vi "FunctionSelector.vi"(4 "System Control In":T2={"Start"=FALSE, "Stop"=FALSE, "Power System Enable"=FALSE, "SSG Control"=FALSE, "Virtual Inertia"=FALSE, "Manual Current"=FALSE, "Discharge"=FALSE, "Spot Generation"=FALSE, "Charge Control"=FALSE, "Watchdog"=FALSE, "ComAp Fault"=FALSE, "Clear Gen Faults"=FALSE, "Clear PV Faults"=FALSE, "Clear System Faults"=FALSE, "Clear PC Faults"=FALSE, "Clear ES Faults"=FALSE, "Clear Watchdog Faults"=FALSE, "PS V Setpoint"=0.0, "Manual Current"=0.0, "CC V Setpoint"=0.0, "Gen Capacity"=0.0, "Gen Reserve"=0.0, "VI gain P"=0.0, "CC gain P"=0.0, "Nom Hz"=0.0, "Spot Gen Op Value"=50.0, "CC gain I"=0.0, "CC Charge"=100.0, "CC Discharge"=-100.0, "Discharge Current"=-25.0, "Sign Of Life"=FALSE, "Reverse Rotation"=FALSE, "String Selector"=enum."3 Strings"}, 5 "Current Limit Parameters In":T4, 6 "Error In":errorcluster, 7 "FPGA Data":T1, 8 "VI Current In":dbl, 9 "CC Current In":dbl) -> (0 "Error Out":errorcluster, 2 "Current Out":dbl)   [LabVIEW 2013]
uses:
  eng/trunk/ni/cRIO Master Files/Controls/CurrentLimitParameters.ctl
  eng/trunk/ni/cRIO Master Files/Controls/SystemControl.ctl
  eng/trunk/ni/cRIO Master Files/Controls/StringSelector.ctl
  Controls/FPGAData.ctl
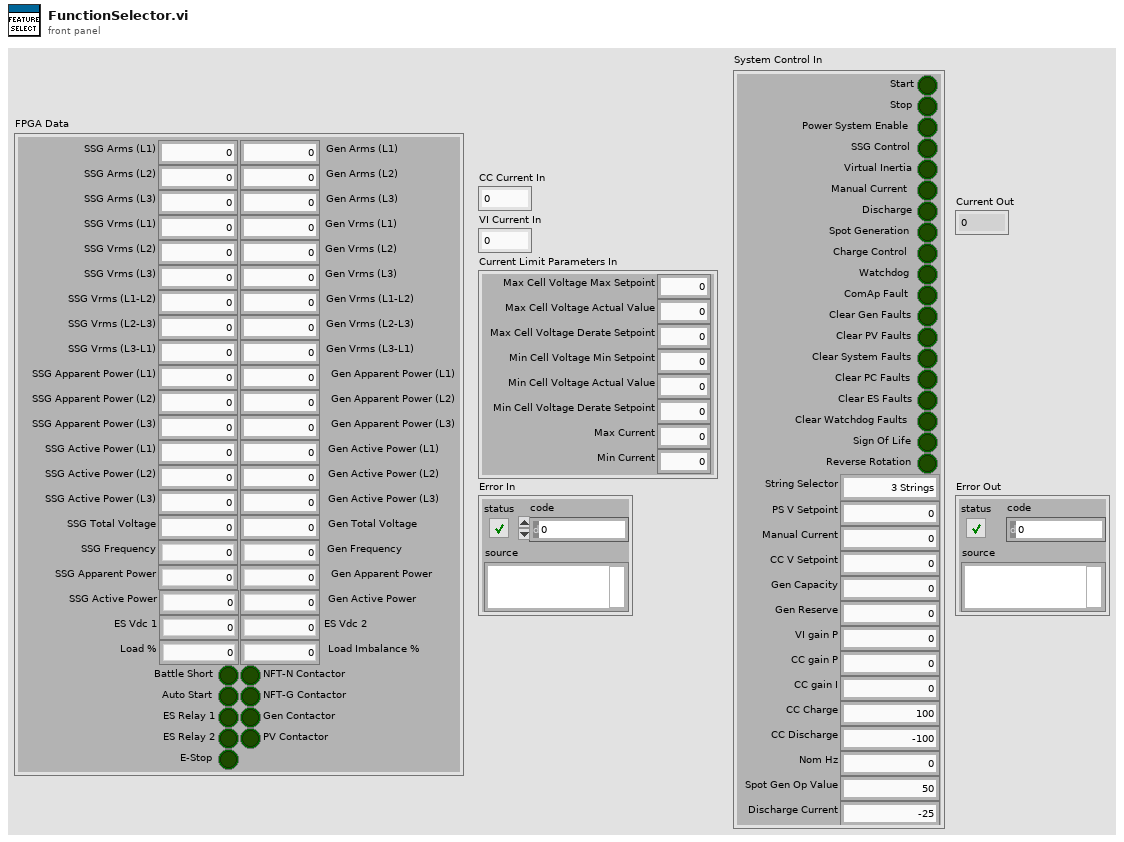
[diagram p1: front panel]
types:
  T1 = typedef "FPGAData.ctl" = cluster{"SSG Frequency":sgl, "SSG Total Voltage":dbl, "SSG Active Power":sgl, "SSG Apparent Power":sgl, "SSG Active Power (L1)":dbl, "SSG Active Power (L2)":dbl, "SSG Active Power (L3)":dbl, "SSG Apparent Power (L1)":dbl, "SSG Apparent Power (L2)":dbl, "SSG Apparent Power (L3)":dbl, "SSG Vrms (L1-L2)":dbl, "SSG Vrms (L2-L3)":dbl, "SSG Vrms (L3-L1)":dbl, "SSG Vrms (L1)":dbl, "SSG Vrms (L2)":dbl, "SSG Vrms (L3)":dbl, "SSG Arms (L1)":dbl, "SSG Arms (L2)":dbl, "SSG Arms (L3)":dbl, "Gen Frequency":sgl, "Gen Total Voltage":dbl, "Gen Active Power":sgl, "Gen Apparent Power":sgl, "Gen Active Power (L1)":dbl, "Gen Active Power (L2)":dbl, "Gen Active Power (L3)":dbl, "Gen Apparent Power (L1)":dbl, "Gen Apparent Power (L2)":dbl, "Gen Apparent Power (L3)":dbl, "Gen Vrms (L1-L2)":dbl, "Gen Vrms (L2-L3)":dbl, "Gen Vrms (L3-L1)":dbl, "Gen Vrms (L1)":dbl, "Gen Vrms (L2)":dbl, "Gen Vrms (L3)":dbl, "Gen Arms (L1)":dbl, "Gen Arms (L2)":dbl, "Gen Arms (L3)":dbl, "ES Vdc 1":sgl, "ES Vdc 2":sgl, "Load %":sgl, "Load Imbalance %":sgl, "E-Stop":bool, "Battle Short":bool, "Auto Start":bool, "Gen Contactor":bool, "ES Relay 1":bool, "ES Relay 2":bool, "NFT-N Contactor":bool, "NFT-G Contactor ":bool, "PV Contactor":bool}
  T2 = typedef "SystemControl.ctl" = cluster{"Start":bool, "Stop":bool, "Power System Enable":bool, "SSG Control":bool, "Virtual Inertia":bool, "Manual Current":bool, "Discharge":bool, "Spot Generation":bool, "Charge Control":bool, "Watchdog":bool, "ComAp Fault":bool, "Clear Gen Faults":bool, "Clear PV Faults":bool, "Clear System Faults":bool, "Clear PC Faults":bool, "Clear ES Faults":bool, "Clear Watchdog Faults":bool, "PS V Setpoint":dbl, "Manual Current":dbl, "CC V Setpoint":dbl, "Gen Capacity":dbl, "Gen Reserve":dbl, "VI gain P":dbl, "CC gain P":dbl, "Nom Hz":dbl, "Spot Gen Op Value":dbl, "CC gain I":dbl, "CC Charge":dbl, "CC Discharge":dbl, "Discharge Current":dbl, "Sign Of Life":bool, "Reverse Rotation":bool, "String Selector":T3}
  T3 = typedef "StringSelector.ctl" = enum16{"1 String (1)", "1 String (2)", "1 String (3)", "2 Strings (1, 2)", "2 Strings (2, 3)", "2 Strings (1, 3)", "3 Strings"}
  T4 = typedef "CurrentLimitParameters.ctl" = cluster{"Max Cell Voltage Max Setpoint":dbl, "Max Cell Voltage Actual Value":dbl, "Max Cell Voltage Derate Setpoint":dbl, "Min Cell Voltage Min Setpoint":dbl, "Min Cell Voltage Actual Value":dbl, "Min Cell Voltage Derate Setpoint":dbl, "Max Current":dbl, "Min Current":dbl}
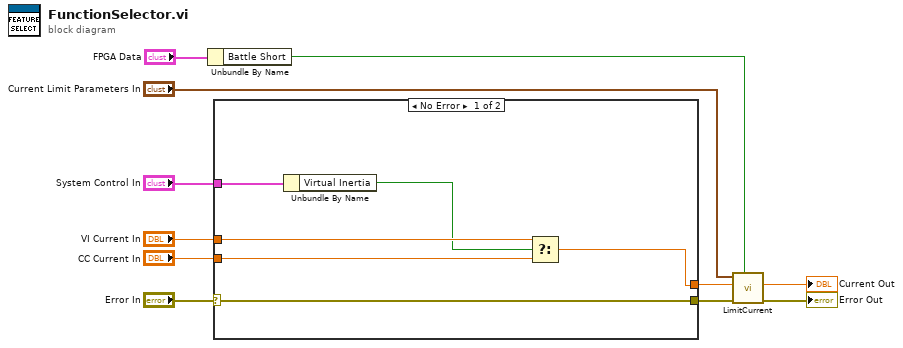
[diagram p0: block diagram]
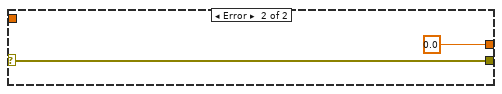
[diagram p2: hidden frame]
diagram:
  n1 = Unbundle By Name("FPGA Data") -> ("Battle Short"=w1:bool)
  n2 = case shown="No Error" "Error In" {
    selector: "Error In" -> [w17 w19]
    tunnel: "CC Current In" -> [w13 _]
    tunnel: "VI Current In" -> [w15 _]
    tunnel: [w17 w19] -> w7
    tunnel: [w12 0.0] -> w4
    tunnel: "System Control In" -> [w16 _]
    frame No Error {
      n3 = Unbundle By Name(w16) -> ("Virtual Inertia"=w14:bool)
      n4 = Select(t=w15, s=w14, f=w13) -> (s? t:f=w12:dbl)
    }
    frame Error {
    }
  }
  n5 = call "LimitCurrent.vi"("Battle Short"=w1, "Error In"=w7, "Current In"=w4, "Current Limit Parameters"="Current Limit Parameters In") -> ("Error Out"=→"Error Out":errorcluster, "Current Out"=→"Current Out":dbl)  [unwired: 3 in, 1 out]
